vi "nanomsg_get_monitor.vi"(6 "error in":errorcluster, 9 "monitor in":refnum<class "nanomsg_socket.lvclass">) -> (0 "error out":errorcluster, 2 "event":T1, 3 "monitor out":refnum<class "nanomsg_socket.lvclass">, 4 "addr":string, 5 "value":i32)   [LabVIEW 2014, in "nanomsg.lvlib" / "nanomsg_socket.lvclass"]
doc: "Receive a montor message from the provided socket and decodes it into readable form. The type of the event, associated endpoint address, and event-specific integer are returned.\n\nThis is a blocking call, and will terminate with the monitor socket.\n\nDetails on the event data: http://api.zeromq.org/3-2:zmq-socket-monitor"
uses:
  nanomsg_socket.lvclass
  monitor_event.ctl
  nanomsg_socket.lvclass/nanomsg_socket.ctl
  <vilib>/Utility/error.llb/Error Cluster From Error Code.vi
  nanomsg.lvlib
panel:
  # "NN"
  # "labview"
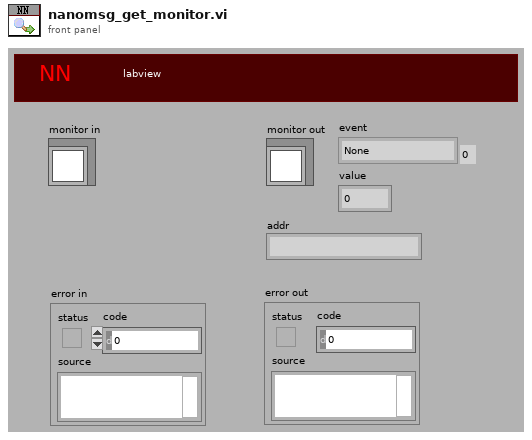
[diagram p1: front panel]
types:
  T1 = typedef "nanomsg.lvlib/monitor_event.ctl" = enum8{"None", "Connected", "Connect Delayed", "Connect Retry", "Listening", "Bind Failed", "Accepted", "Accept Failed", "Closed", "Close Failed", "Disconnected"}
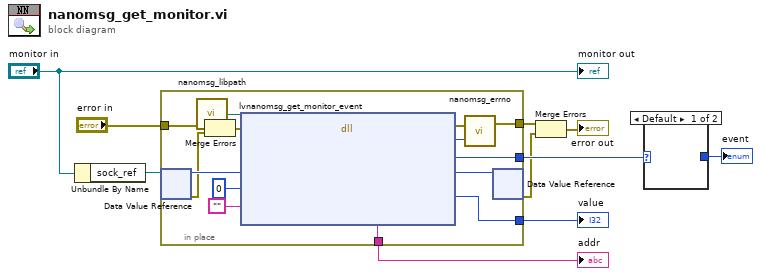
[diagram p0: block diagram]
diagram:
  n1 = Unbundle By Name("monitor in") -> ("sock_ref"=w8:refnum<data-value>)
  n2 = in-place {
    in-place-border: "error in" -> [w22]
    in-place-border: [w21] -> w3
    in-place-border: [w20] -> w6
    in-place-border: [w14] -> w5
    in-place-border: [w13] -> w7
    n3 = in-place-dvr #1(w8) -> (w19:u64, w11:errorcluster)
    n4 = call "nanomsg_libpath.vi"() -> ("path"=w17:path)
    n5 = Merge Errors(w22, w11) -> (w12:errorcluster)
    n6 = dll-call lib="?" fn="lvnanomsg_get_monitor_event" ("zmq_labview.dll:lvzmq_socket")(path in=w17, error in=w12, "sock_obj"=w19, "intval"=0, "addr"="") -> (error out=w23:errorcluster, "return type"=w14:i32, "sock_obj"=w18:u64, "intval"=w13:i32, "addr"=w20:string)  [unwired: 3 in, 1 out]
    n7 = call "nanomsg_errno.vi"("retval"=w14, "error in"=w23) -> ("error out"=w21:errorcluster)  [unwired: 1 out]
    n8 = in-place-dvr #1(w18) -> (w2:errorcluster)  [unwired: 1 out]
  }
  "addr" <- w6
  "value" <- w7
  n9 = Merge Errors(w3, w2) -> (→"error out":errorcluster)
  n10 = case shown="Default" w5 {
    selector: w5 -> [_ w24]
    tunnel: [_ w24] -> w4
    frame Default {
    }
    frame 1..10 {
    }
  }
  "event" <- w4
  "monitor out" <- "monitor in"
